vi "autofocus-main.vi"() -> ()   [LabVIEW 2014]
uses:
  Shutter Control/Shutter SubVis/user event shutter global.ctl
  Stage Control/Stage SubVis/move stage.ctl
  autofocus-globals.vi
  tirf-lock-globals.vi
  <vilib>/Analysis/polynomials.llb/1D Polynomial Evaluation (DBL).vi
  <vilib>/Analysis/NI_AALPro.lvlib
panel:
  out "delta Z":dbl format="%#_13g"
  out "Calibration curve and fit":cluster{"z (um)":ext[], "QPD position":dbl[]}[](graph)
  out "Power":dbl format="%#_13g"
  out "Error Out":errorcluster
  in  "Error In":errorcluster
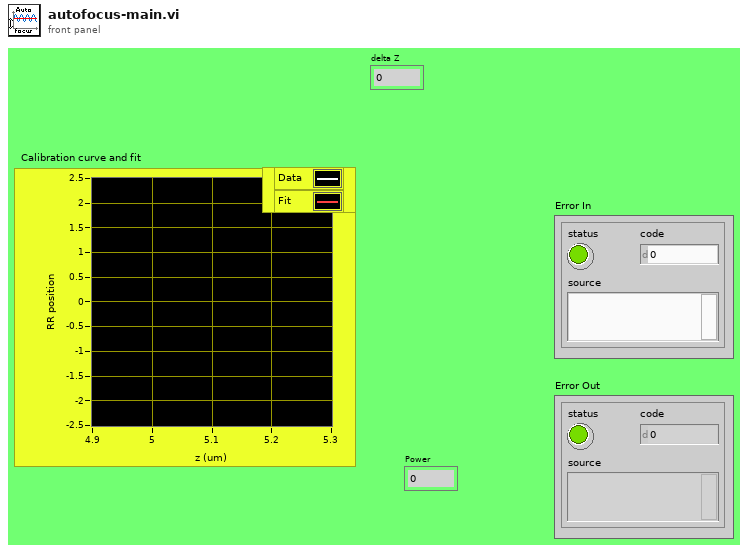
[diagram p1: front panel]
types:
  T1 = typedef "user event shutter global.ctl" = cluster{"Camera Shutter":bool, "Wheel Speed":u8, "Laser Shutter":enum32{"No Selection", "GFP", "Cy3 Long \nPass", "Cy3", "Cy5", "Off", "IR"}}
  T2 = enum32{"No Selection", "GFP", "Cy3 Long \nPass", "Cy3", "Cy5", "Off", "IR"}
  T3 = typedef "move stage.ctl" = cluster{"dx (um) (0 -> ignore)":ext, "dy (um) (0 -> ignore)":ext, "dz (um) (0 -> ignore)":ext, "Re-center x,y":bool, "Re-center z":bool, "x (um) (-1 -> ignore)":dbl, "y (um) (-1 -> ignore)":dbl, "z (um) (-1 -> ignore)":dbl}
  T4 = cluster{"Best Polynomial Fit":dbl[], "QPD position":dbl[]}
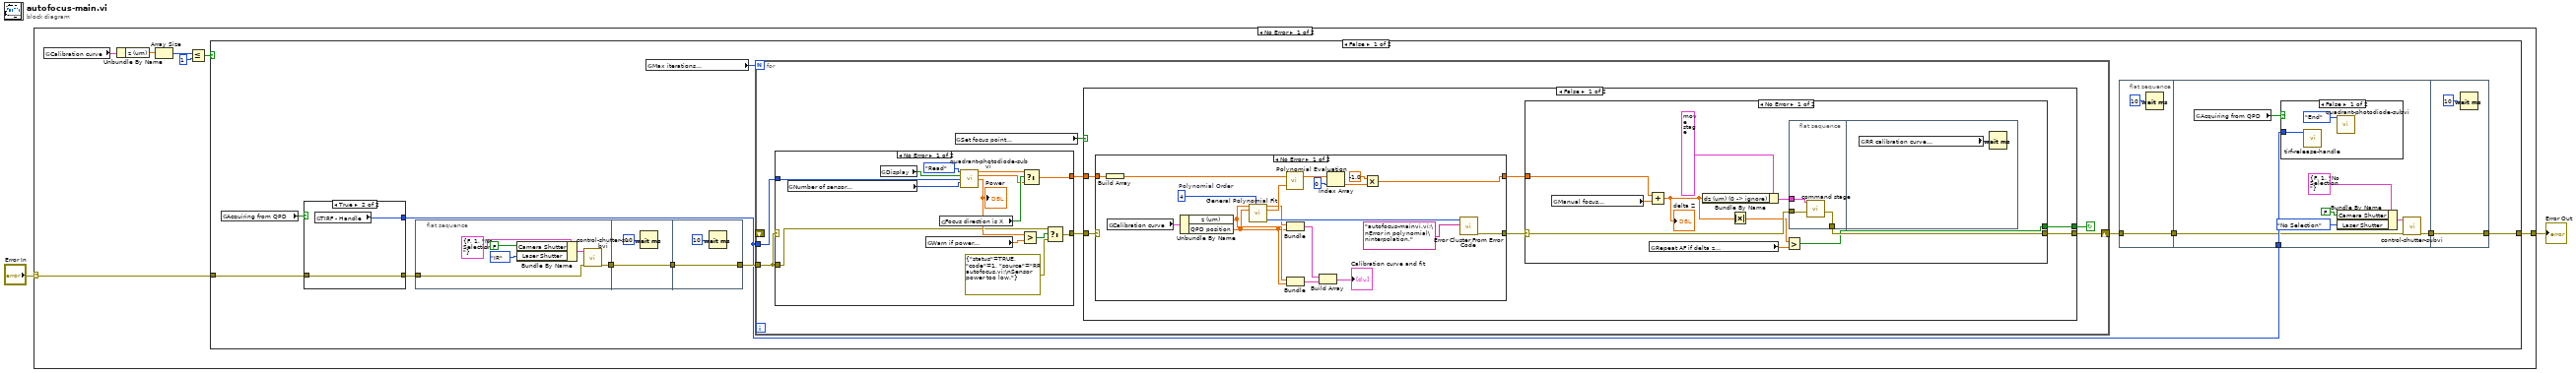
[diagram p0: block diagram]
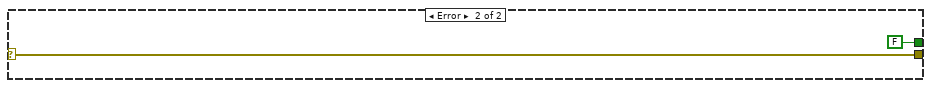
[diagram p3: hidden frame]
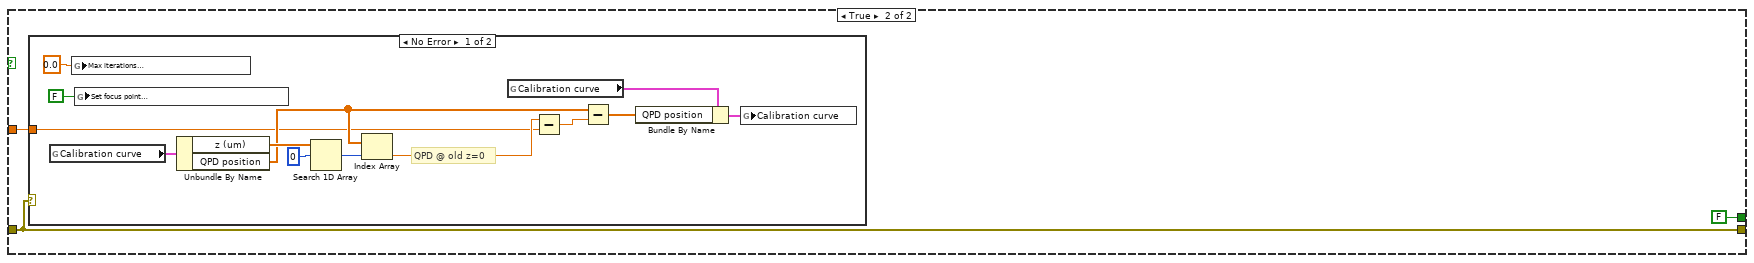
[diagram p5: hidden frame]
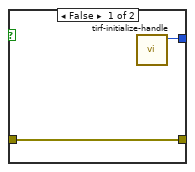
[diagram p8: hidden frame]
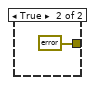
[diagram p9: hidden frame]
diagram:
  n1 = case shown="No Error" "Error In" {
    selector: "Error In" -> [w4 w132]
    tunnel: [w3 w132] -> w1
    frame No Error {
      n2 = global read "autofocus-globals.vi" "Calibration curve"() -> (w9:cluster{"z (um)":ext[], "QPD position":dbl[]})
      n3 = Unbundle By Name(w9) -> ("z (um)"=w6:ext[])
      n4 = Array Size(array=w6) -> (size(s)=w5:i32)
      n5 = Less Or Equal?(x=w5, y=1) -> (x <= y?=w7:bool)
      n6 = case shown="False" w7 {
        tunnel: w4 -> [w21 _]
        tunnel: [w12 errorcluster {"status"=TRUE, "code"=1, "source"="RR autofocus.vi:\nCan't autofocus because no\nautofocus calibration curve has been stored."} ("f")] -> w3
        frame False {
          n7 = global read "autofocus-globals.vi" "Acquiring from QPD"() -> (w20:bool)
          n8 = case shown="True" w20 {
            tunnel: w21 -> [w128 w130]
            tunnel: [w128 w130] -> w19
            tunnel: [w127 w129] -> w11
            frame False {
              n9 = call "tirf-initialize-handle.vi"() -> ("handle"=w127:i32)  [unwired: 11 in]
            }
            frame True {
              n10 = global read "autofocus-globals.vi" "TIRF - Handle"() -> (w129:u32)
            }
          }
          n11 = flat-sequence {
            tunnel: [w121] -> w18
            tunnel: w19 -> [w122]
            tunnel: w18 -> [w123]
            tunnel: [w123] -> w10
            tunnel: [w125] -> w16
            tunnel: w10 -> [w125]
            frame #0 {
              n12 = Bundle By Name(cluster=T1 {"Camera Shutter"=FALSE, "Wheel Speed"=1, "Laser Shutter"=enum."No Selection"} ("Shutter Control"), "Camera Shutter"=FALSE, "Laser Shutter"=T2."IR") -> (w118:T1)
              n13 = call "control-shutter-subvi.vi"("Error In"=w122, "Shutter Control"=w118) -> ("Error Out"=w121:errorcluster)  [unwired: 9 in]
            }
            frame #1 {
              n14 = Wait (ms)(milliseconds to wait=u32 10) -> ()  [unwired: 1 out]
            }
            frame #2 {
              n15 = Wait (ms)(milliseconds to wait=u32 10) -> ()  [unwired: 1 out]
            }
          }
          n16 = global read "autofocus-globals.vi" "Max iterations \nper autofocus"() -> (w17:i32)
          n17 = for {
            N: w17 -> [_]
            tunnel: w16 -> [w36]
            shift-right: [w38] -> w15
            shift-left: _ -> [_]
            tunnel: w11 -> [w37]
            stop <- w39 continue-if-true
            n18 = case shown="No Error" w36 {
              selector: w36 -> [_ w116]
              tunnel: [w107 w116] -> w42
              tunnel: [w106 _] -> w40
              tunnel: w37 -> [w105 _]
              tunnel: w36 -> [w102 _]
              frame No Error {
                n19 = global read "autofocus-globals.vi" "Number of sensor\nreadings to average"() -> (w104:i32)
                n20 = global read "tirf-lock-globals.vi" "Display"() -> (w103:bool)
                n21 = global read "autofocus-globals.vi" "Warn if power \nless than"() -> (w109:dbl)
                n22 = global read "autofocus-globals.vi" "Focus direction is X"() -> (w114:bool)
                n23 = call "quadrant-photodiode-subvi.vi"("Mode"=enum16{"Start", "Read", "End"}."Read", "Display"=w103, "Handle"=w105, "Averages"=w104) -> ("coerced(x)"=w112:dbl, "coerced(y)"=w113:dbl, "Power (mw)"=w108:dbl)  [unwired: 9 in]
                "Power" <- w108
                n24 = Greater?(x=w108, y=w109) -> (0:w110:bool)
                n25 = Select(t=w112, s=w114, f=w113) -> (s? t:f=w106:dbl)
                n26 = Select(t=w102, s=w110, f=errorcluster {"status"=TRUE, "code"=1, "source"="RR autofocus.vi:\nSensor power too low."}) -> (s? t:f=w107:errorcluster)
              }
              frame Error {
              }
            }
            n27 = global read "autofocus-globals.vi" "Set focus point\nto current z position"() -> (w41:bool)
            n28 = case shown="False" w41 {
              tunnel: w42 -> [w48 w86]
              tunnel: w40 -> [w46 w87]
              tunnel: [w44 FALSE] -> w39
              tunnel: [w43 w86] -> w38
              frame False {
                n29 = case shown="No Error" w48 {
                  selector: w48 -> [_ w85]
                  tunnel: [w78 w85] -> w47
                  tunnel: w46 -> [w83 w84]
                  tunnel: [w74 w84] -> w45
                  frame No Error {
                    w81 = 4  # Polynomial Order
                    n30 = Build Array(w83) -> (w69:dbl[])
                    n31 = global read "autofocus-globals.vi" "Calibration curve"() -> (w82:cluster{"z (um)":ext[], "QPD position":dbl[]})
                    n32 = Unbundle By Name(w82) -> ("z (um)"=w66:ext[], "QPD position"=w65:dbl[])
                    n33 = call <vilib>:"General Polynomial Fit.vi"("Y"=w66, "polynomial order"=w81, "X"=w65) -> ("Best Polynomial Fit"=w67:dbl[], "Polynomial Coefficients"=w70:dbl[], "error"=w79:i32)  [unwired: 9 in, 1 out]
                    n34 = call-poly <vilib>:"Polynomial Evaluation.vi"("P(x)"=w70, "A"=w69) -> ("P(A)"=w68:dbl[])  [unwired: 1 out]
                    n35 = Bundle("Best Polynomial Fit"=w67, "QPD position"=w65) -> (w73:T4)  [unwired: 1 in]
                    n36 = Bundle("z (um)"=w66, "QPD position"=w65) -> (w72:cluster{"z (um)":ext[], "QPD position":dbl[]})  [unwired: 1 in]
                    n37 = Build Array(w73, w72) -> (→"Calibration curve and fit":cluster{"z (um)":ext[], "QPD position":dbl[]}[])
                    n38 = Index Array(array=w68, index=0) -> (element=w76:dbl)
                    n39 = Multiply(x=-1.0, y=w76) -> (x*y=w74:dbl)
                    n40 = call <vilib>:"Error Cluster From Error Code.vi"("error message (\"\")"="autofocus-mainvi.vi:\nError in polynomial\ninterpolation." ("error message (\"\")"), "error code (0)"=w79) -> ("error out"=w78:errorcluster)  [unwired: 2 in, 5 out]
                  }
                  frame Error {
                  }
                }
                n41 = case shown="No Error" w47 {
                  selector: w47 -> [w58 w64]
                  tunnel: [w57 w64] -> w43
                  tunnel: w45 -> [w55 _]
                  tunnel: [w49 FALSE] -> w44
                  frame No Error {
                    n42 = global read "autofocus-globals.vi" "Manual focus\noffset (um)"() -> (w56:dbl)
                    n43 = Add(x=w55, y=w56) -> (x+y=w52:dbl)
                    "delta Z" <- w52
                    n44 = global read "autofocus-globals.vi" "Repeat AF if delta z \ngreater than (um)"() -> (w50:dbl)
                    n45 = Bundle By Name(cluster=T3 {"dx (um) (0 -> ignore)"=0.0, "dy (um) (0 -> ignore)"=0.0, "dz (um) (0 -> ignore)"=0.0, "Re-center x,y"=FALSE, "Re-center z"=FALSE, "x (um) (-1 -> ignore)"=-1.0, "y (um) (-1 -> ignore)"=-1.0, "z (um) (-1 -> ignore)"=-1.0} ("Command Stage"), "dz (um) (0 -> ignore)"=w52) -> (w53:T3)
                    n46 = Absolute Value(x=w52) -> (abs(x)=w51:dbl)
                    n47 = Greater?(x=w51, y=w50) -> (0:w49:bool)
                    n48 = flat-sequence {
                      tunnel: w58 -> [w61]
                      tunnel: [w60] -> w57
                      tunnel: w53 -> [w59]
                      frame #0 {
                        n49 = call "command stage.vi"("Error In"=w61, "Command Stage"=w59) -> ("Error Out"=w60:errorcluster)  [unwired: 9 in]
                      }
                      frame #1 {
                        n50 = global read "autofocus-globals.vi" "RR calibration curve\nsettle time (ms)"() -> (w62:u16)
                        n51 = Wait (ms)(milliseconds to wait=w62) -> ()  [unwired: 1 out]
                      }
                    }
                  }
                  frame Error {
                  }
                }
              }
              frame True {
                n52 = case shown="No Error" w86 {
                  tunnel: w87 -> [w94 _]
                  frame No Error {
                    # "QPD @ old z=0"
                    n53 = global read "autofocus-globals.vi" "Calibration curve"() -> (w101:cluster{"z (um)":ext[], "QPD position":dbl[]})
                    n54 = global write "autofocus-globals.vi" "Max iterations \nper autofocus"(0.0) -> ()
                    n55 = global write "autofocus-globals.vi" "Set focus point\nto current z position"(FALSE) -> ()
                    n56 = Unbundle By Name(w101) -> ("z (um)"=w99:ext[], "QPD position"=w95:dbl[])
                    n57 = Search 1D Array(1D array=w99, element=0) -> (index of element=w100:i32)  [unwired: 1 in]
                    n58 = Index Array(array=w95, index=w100) -> (element=w97:dbl)
                    n59 = global read "autofocus-globals.vi" "Calibration curve"() -> (w93:cluster{"z (um)":ext[], "QPD position":dbl[]})
                    n60 = Subtract(x=w97, y=w94) -> (x-y=w96:dbl)
                    n61 = Subtract(x=w95, y=w96) -> (x-y=w92:dbl[])
                    n62 = Bundle By Name(cluster=w93, "QPD position"=w92) -> (w91:cluster{"z (um)":ext[], "QPD position":dbl[]})
                    n63 = global write "autofocus-globals.vi" "Calibration curve"(w91) -> ()
                  }
                  frame Error {
                  }
                }
              }
            }
          }
          n64 = flat-sequence {
            tunnel: [w23] -> w13
            tunnel: w15 -> [w23]
            tunnel: [w28] -> w14
            tunnel: w13 -> [w29]
            tunnel: w11 -> [w30]
            tunnel: w14 -> [w35]
            tunnel: [w35] -> w12
            frame #0 {
              n65 = Wait (ms)(milliseconds to wait=u32 10) -> ()  [unwired: 1 out]
            }
            frame #1 {
              n66 = global read "autofocus-globals.vi" "Acquiring from QPD"() -> (w31:bool)
              n67 = case shown="False" w31 {
                tunnel: w30 -> [w32 _]
                frame False {
                  n68 = call "tirf-release-handle.vi"("handle"=w32) -> ()  [unwired: 11 in]
                  n69 = call "quadrant-photodiode-subvi.vi"("Mode"=enum16{"Start", "Read", "End"}."End") -> ()  [unwired: 12 in, 3 out]
                }
                frame True {
                }
              }
              n70 = Bundle By Name(cluster=T1 {"Camera Shutter"=FALSE, "Wheel Speed"=1, "Laser Shutter"=enum."No Selection"} ("Shutter Control"), "Camera Shutter"=FALSE, "Laser Shutter"=T2."No Selection") -> (w24:T1)
              n71 = call "control-shutter-subvi.vi"("Error In"=w29, "Shutter Control"=w24) -> ("Error Out"=w28:errorcluster)  [unwired: 9 in]
            }
            frame #2 {
              n72 = Wait (ms)(milliseconds to wait=u32 10) -> ()  [unwired: 1 out]
            }
          }
        }
        frame True {
        }
      }
    }
    frame Error {
    }
  }
  "Error Out" <- w1
